vi "sub-make menu text.vi"(11 "languages":T1(array[cluster])) -> (3 "menu text":string)   [LabVIEW 2011]
uses:
  sub-Language global.vi
  sub-Language-get str-const.vi
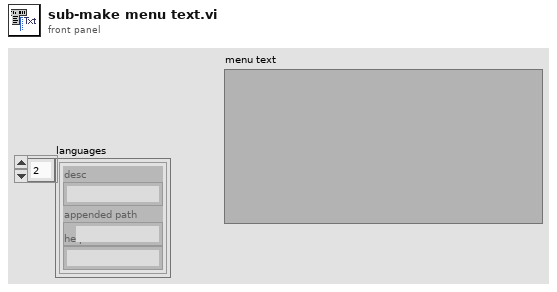
[diagram p1: front panel]
types:
  T1 = cluster{"desc":string, "appended path":path, "help dir":string}[]
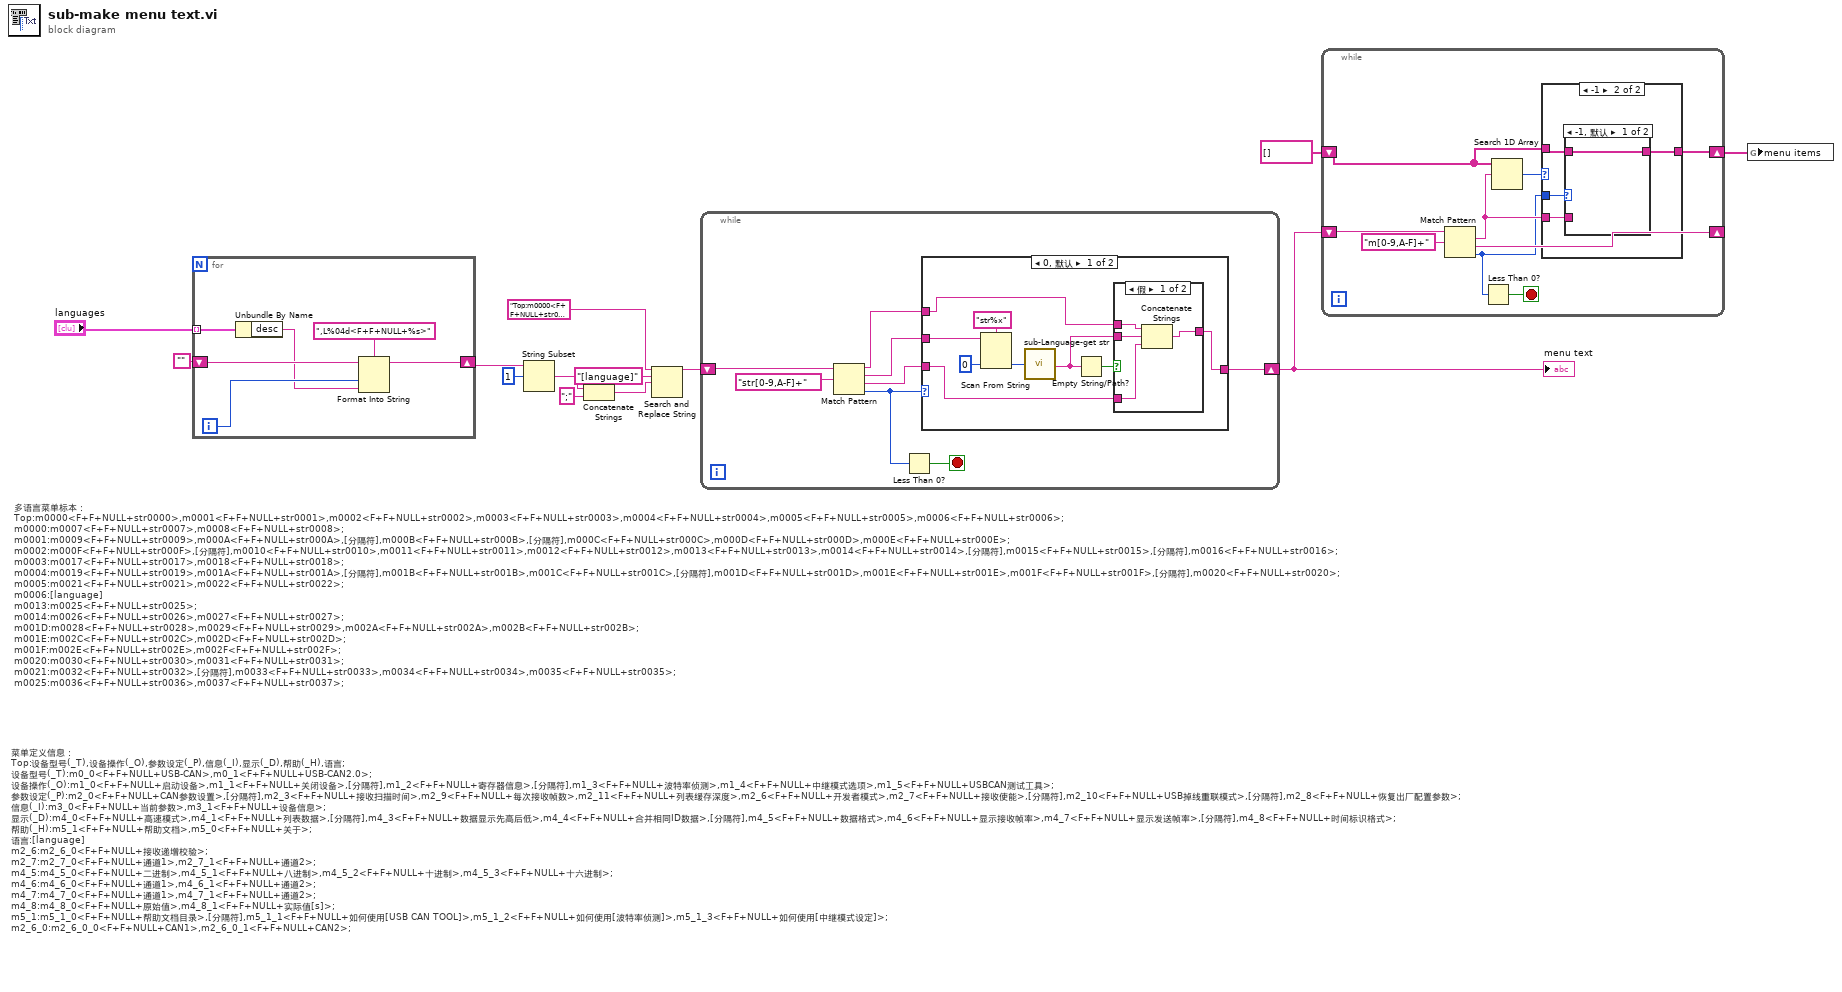
[diagram p0: block diagram]
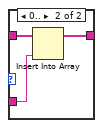
[diagram p3: hidden frame]
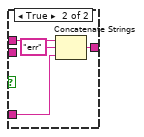
[diagram p4: hidden frame]
diagram:
  # "菜单定义信息：\nTop:设备型号(_T),设备操作(_O),参数设定(_P),信息(_I),显示(_D),帮助(_H),语言;\n设备型号(_T):m0_0<F+F+NULL+USB-CAN>,m0_1<F+F+NULL+USB-CAN2.0>;\n设备操作(_O):m1_0<F+F+NULL+启动设备>,m1_1<F+F+NULL+关闭设备>,[分隔符],m1_2<F+F+NULL+寄存器信息>,[分隔符],m1_3<F+F+NULL+波特率侦测>,m1_4<F+F+NULL+中继模式选项>,m1_5<F+F+NULL+USBCAN测试工具>;\n参数设定(_P):m2_0<F+F+NULL+CAN参数设置>,[分隔符],m2_3<F+F+NULL+接收扫描时间>,m2_9<F+F+NULL+每次接收帧数>,m2_11<F+F+NULL+列表缓存深度>,m2_6<F+F+NULL+开发者模式>,m2_7<F+F+NULL+接收使能>,[分隔符],m2_10<F+F+NULL+USB掉线重联模式>,[分隔符],m2_8<F+F+NULL+恢复出厂配置参数>;\n信息(_I):m3_0<F+F+NULL+当前参数>,m3_1<F+F+NULL+设备信息>;\n显示(_D):m4_0<F+F+NULL+高速模式>,m4_1<F+F+NULL+列表数据>,[分隔符],m4_3<F+F+NULL+数据显示先高后低>,m4_4<F+F+NULL+合并相同ID数据>,[分隔符],m4_5<F+F+NULL+数据格式>,m4_6<F+F+NULL+显示接收帧率>,m4_7<F+F+NULL+显示发送帧率>,[分隔符],m4_8<F+F+NULL+时间标识格式>;\n帮助(_H):m5_1<F+F+NULL+帮助文档>,m5_0<F+F+NULL+关于>;\n语言:[language]\nm2_6:m2_6_0<F+F+NULL+接收递增校验>;\nm2_7:m2_7_0<F+F+NULL+通道1>,m2_7_1<F+F+NULL+通道2>;\nm4_5:m4_5_0<F+F+NULL+二进制>,m4_5_1<F+F+NULL+八进制>,m4_5_2<F+F+NULL+十进制>,m4_5_3<F+F+NULL+十六进制>;\nm4_6:m4_6_0<F+F+NULL+通道1>,m4_6_1<F+F+NULL+通道2>;\nm4_7:m4_7_0<F+F+NULL+通道1>,m4_7_1<F+F+NULL+通道2>;\nm4_8:m4_8_0<F+F+NULL+原始值>,m4_8_1<F+F+NULL+实际值[s]>;\nm5_1:m5_1_0<F+F+NULL+帮助文档目录>,[分隔符],m5_1_1<F+F+NULL+如何使用[USB CAN TOOL]>,m5_1_2<F+F+NULL+如何使用[波特率侦测]>,m5_1_3<F+F+NULL+如何使用[中继模式设定]>;\nm2_6_0:m2_6_0_0<F+F+NULL+CAN1>,m2_6_0_1<F+F+NULL+CAN2>;"
  # "多语言菜单标本：\nTop:m0000<F+F+NULL+str0000>,m0001<F+F+NULL+str0001>,m0002<F+F+NULL+str0002>,m0003<F+F+NULL+str0003>,m0004<F+F+NULL+str0004>,m0005<F+F+NULL+str0005>,m0006<F+F+NULL+str0006>;\nm0000:m0007<F+F+NULL+str0007>,m0008<F+F+NULL+str0008>;\nm0001:m0009<F+F+NULL+str0009>,m000A<F+F+NULL+str000A>,[分隔符],m000B<F+F+NULL+str000B>,[分隔符],m000C<F+F+NULL+str000C>,m000D<F+F+NULL+str000D>,m000E<F+F+NULL+str000E>;\nm0002:m000F<F+F+NULL+str000F>,[分隔符],m0010<F+F+NULL+str0010>,m0011<F+F+NULL+str0011>,m0012<F+F+NULL+str0012>,m0013<F+F+NULL+str0013>,m0014<F+F+NULL+str0014>,[分隔符],m0015<F+F+NULL+str0015>,[分隔符],m0016<F+F+NULL+str0016>;\nm0003:m0017<F+F+NULL+str0017>,m0018<F+F+NULL+str0018>;\nm0004:m0019<F+F+NULL+str0019>,m001A<F+F+NULL+str001A>,[分隔符],m001B<F+F+NULL+str001B>,m001C<F+F+NULL+str001C>,[分隔符],m001D<F+F+NULL+str001D>,m001E<F+F+NULL+str001E>,m001F<F+F+NULL+str001F>,[分隔符],m0020<F+F+NULL+str0020>;\nm0005:m0021<F+F+NULL+str0021>,m0022<F+F+NULL+str0022>;\nm0006:[language]\nm0013:m0025<F+F+NULL+str0025>;\nm0014:m0026<F+F+NULL+str0026>,m0027<F+F+NULL+str0027>;\nm001D:m0028<F+F+NULL+str0028>,m0029<F+F+NULL+str0029>,m002A<F+F+NULL+str002A>,m002B<F+F+NULL+str002B>;\nm001E:m002C<F+F+NULL+str002C>,m002D<F+F+NULL+str002D>;\nm001F:m002E<F+F+NULL+str002E>,m002F<F+F+NULL+str002F>;\nm0020:m0030<F+F+NULL+str0030>,m0031<F+F+NULL+str0031>;\nm0021:m0032<F+F+NULL+str0032>,[分隔符],m0033<F+F+NULL+str0033>,m0034<F+F+NULL+str0034>,m0035<F+F+NULL+str0035>;\nm0025:m0036<F+F+NULL+str0036>,m0037<F+F+NULL+str0037>;"
  n1 = for {
    tunnel: "languages" -> [w19] mode=indexing
    shift-right: [w14] -> w12
    shift-left: "" -> [w18]
    i -> [w16]
    n2 = Unbundle By Name(w19) -> ("desc"=w15:string)
    n3 = Format Into String(format string=",L%04d<F+F+NULL+%s>" ("格式字符串"), initial string=w18, w16, w15) -> (resulting string=w14:string)  [unwired: 1 in, 1 out]
  }
  n4 = String Subset(string=w12, offset (0)=1 ("偏移量(0)")) -> (substring=w10:string)  [unwired: 1 in]
  n5 = Concatenate Strings(w10, ";" ("字符串")) -> (w7:string)
  n6 = Search and Replace String(input string="Top:m0000<F+F+NULL+str0000>,m0001<F+F+NULL+str0001>,m0002<F+F+NULL+str0002>,m0003<F+F+NULL+str0003>,m0004<F+F+NULL+str0004>,m0005<F+F+NULL+str0005>,m0006<F+F+NULL+str0006>;\nm0000:m0007<F+F+NULL+str0007>,m0008<F+F+NULL+str0008>;\nm0001:m0009<F+F+NULL+str0009>,m000A<F+F+NULL+str000A>,[分隔符],m000B<F+F+NULL+str000B>,[分隔符],m000C<F+F+NULL+str000C>,m000D<F+F+NULL+str000D>,m000E<F+F+NULL+str000E>;\nm0002:m000F<F+F+NULL+str000F>,[分隔符],m0010<F+F+NULL+str0010>,m0011<F+F+NULL+str0011>,m0012<F+F+NULL+str0012>,m0013<F+F+NULL+str0013>,m0014<F+F+NULL+str0014>,[分隔符],m0015<F+F+NULL+str0015>,[分隔符],m0016<F+F+NULL+str0016>;\nm0003:m0017<F+F+NULL+str0017>,m0018<F+F+NULL+str0018>;\nm0004:m0019<F+F+NULL+str0019>,m001A<F+F+NULL+str001A>,[分隔符],m001B<F+F+NULL+str001B>,m001C<F+F+NULL+str001C>,[分隔符],m001D<F+F+NULL+str001D>,m001E<F+F+NULL+str001E>,m001F<F+F+NULL+str001F>,[分隔符],m0020<F+F+NULL+str0020>;\nm0005:m0021<F+F+NULL+str0021>,m0022<F+F+NULL+str0022>;\nm0006:[language]\nm0013:m0025<F+F+NULL+str0025>;\nm0014:m0026<F+F+NULL+str0026>,m0027<F+F+NULL+str0027>;\nm001D:m0028<F+F+NULL+str0028>,m0029<F+F+NULL+str0029>,m002A<F+F+NULL+str002A>,m002B<F+F+NULL+str002B>;\nm001E:m002C<F+F+NULL+str002C>,m002D<F+F+NULL+str002D>;\nm001F:m002E<F+F+NULL+str002E>,m002F<F+F+NULL+str002F>;\nm0020:m0030<F+F+NULL+str0030>,m0031<F+F+NULL+str0031>;\nm0021:m0032<F+F+NULL+str0032>,[分隔符],m0033<F+F+NULL+str0033>,m0034<F+F+NULL+str0034>,m0035<F+F+NULL+str0035>;\nm0025:m0036<F+F+NULL+str0036>,m0037<F+F+NULL+str0037>;" ("String"), search string="[language]" ("搜索字符串"), replace string=w7) -> (result string=w5:string)  [unwired: 5 in, 3 out]
  n7 = while {
    shift-right: [w22] -> w4
    shift-left: w5 -> [w27]
    stop <- w25 stop-if-true
    n8 = Match Pattern(string=w27, regular expression="str[0-9,A-F]+" ("正则表达式")) -> (before substring=w23:string, match substring=w21:string, after substring=w20:string, offset past match=w24:i32)  [unwired: 1 in]
    n9 = Less Than 0?(x=w24) -> (x < 0?=w25:bool)
    n10 = case shown="0, 默认" w24 {
      tunnel: w23 -> [w31 w45]
      tunnel: [w29 w45] -> w22
      tunnel: w21 -> [w36 _]
      tunnel: w20 -> [w30 _]
      frame 0, Default {
        n11 = Scan From String(format string="str%x" ("格式字符串"), input string=w36, default 1=u32 0 ("默认值 1")) -> (output 1=w33:u32)  [unwired: 2 in, 3 out]
        n12 = call-poly "sub-Language-get str.vi"("sid"=w33) -> ("str"=w28:string)
        n13 = Empty String/Path?(string/path=w28) -> (empty?=w32:bool)
        n14 = case shown="假" w32 {
          tunnel: w31 -> [w40 w44]
          tunnel: w30 -> [w38 w43]
          tunnel: [w37 w41] -> w29
          tunnel: w28 -> [w39 _]
          frame False {
            n15 = Concatenate Strings(w40, w39, w38) -> (w37:string)
          }
          frame True {
            n16 = Concatenate Strings(w44, "err" ("字符串"), w43) -> (w41:string)
          }
        }
      }
      frame -1 {
      }
    }
  }
  "menu text" <- w4
  n17 = while {
    shift-right: [w52] -> _
    shift-left: w4 -> [w54]
    shift-right: [w47] -> w2
    shift-left: string[] [] -> [w49]
    stop <- w51 stop-if-true
    n18 = Match Pattern(string=w54, regular expression="m[0-9,A-F]+" ("正则表达式")) -> (match substring=w48:string, after substring=w52:string, offset past match=w46:i32)  [unwired: 1 in, 1 out]
    n19 = Less Than 0?(x=w46) -> (x < 0?=w51:bool)
    n20 = Search 1D Array(1D array=w49, element=w48) -> (index of element=w50:i32)  [unwired: 1 in]
    n21 = case shown="-1" w50 {
      tunnel: w49 -> [w55 w59]
      tunnel: w48 -> [_ w58]
      tunnel: [w55 w57] -> w47
      tunnel: w46 -> [_ w56]
      frame 0, Default {
      }
      frame -1 {
        n22 = case shown="-1, 默认" w56 {
          tunnel: w59 -> [w60 w63]
          tunnel: w58 -> [_ w62]
          tunnel: [w60 w61] -> w57
          frame -1, Default {
          }
          frame 0.. {
            n23 = Insert Into Array(array=w63, new element=w62) -> (w61:string[])  [unwired: 1 in]
          }
        }
      }
    }
  }
  n24 = global write "sub-Language global.vi" "menu items"(w2) -> ()
